vi "updateRowNumber-BellaAlpha.vi"(4 "LoadOut":refnum<vi>, 6 "Numeric":i32, 8 "modeArray 2":refnum<vi>, 9 "Status 3":refnum<vi>, 10 "Name":refnum<vi>, 11 "Array in":refnum<vi>) -> ()   [LabVIEW 2020]
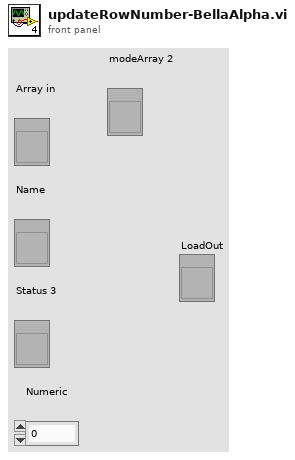
[diagram p1: front panel]
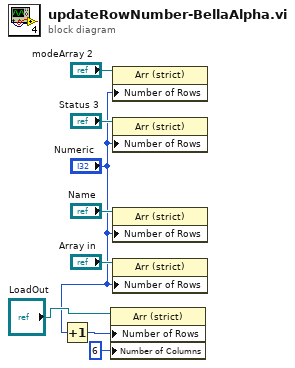
[diagram p0: block diagram]
diagram:
  n1 = Increment(x="Numeric") -> (x+1=w1:i32)
  n2 = property class="Arr (strict)"(reference="LoadOut", "Number of Rows"=w1, "Number of Columns"=u32 6) -> ()  [unwired: 1 in, 2 out]
  n3 = property class="Arr (strict)"(reference="modeArray 2", "Number of Rows"="Numeric") -> ()  [unwired: 1 in, 2 out]
  n4 = property class="Arr (strict)"(reference="Status 3", "Number of Rows"="Numeric") -> ()  [unwired: 1 in, 2 out]
  n5 = property class="Arr (strict)"(reference="Name", "Number of Rows"="Numeric") -> ()  [unwired: 1 in, 2 out]
  n6 = property class="Arr (strict)"(reference="Array in", "Number of Rows"="Numeric") -> ()  [unwired: 1 in, 2 out]
